vi "SendData_Pub.vi"(8 "error in (no error)":errorcluster, 9 "argument list in":T1[](array[typedef]), 11 "LabVIEW-Python-Interface in":refnum<class "PyLVi.lvclass">) -> (0 "error out":errorcluster, 3 "LabVIEW-Python-Interface out":refnum<class "PyLVi.lvclass">)   [LabVIEW 2016, in "PyLVi.lvlib" / "PyLVi.lvclass"]
uses:
  PyLVi.lvclass
  Controls/ArgumentStructure.ctl
  Controls/DescriptorStructure.ctl
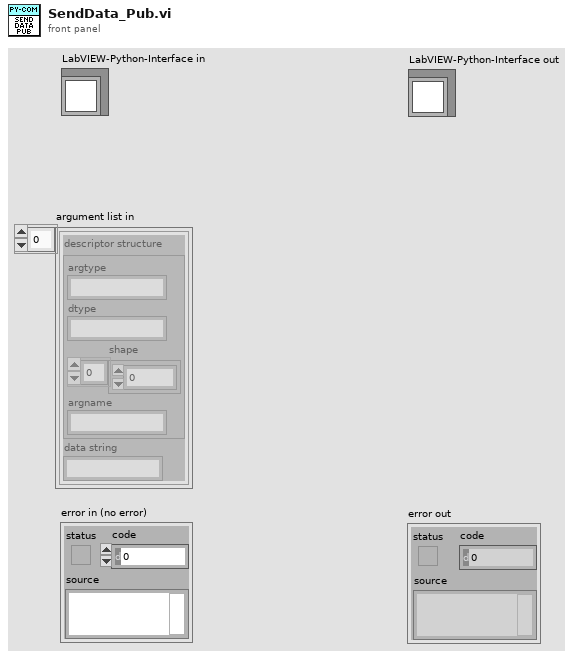
[diagram p1: front panel]
types:
  T1 = typedef "PyLVi.lvlib/PyLVi.lvclass/ArgumentStructure.ctl" = cluster{"descriptor structure":T2, "data string":string}
  T2 = typedef "PyLVi.lvlib/PyLVi.lvclass/DescriptorStructure.ctl" = cluster{"argtype":string, "dtype":string, "shape":u32[], "argname":string}
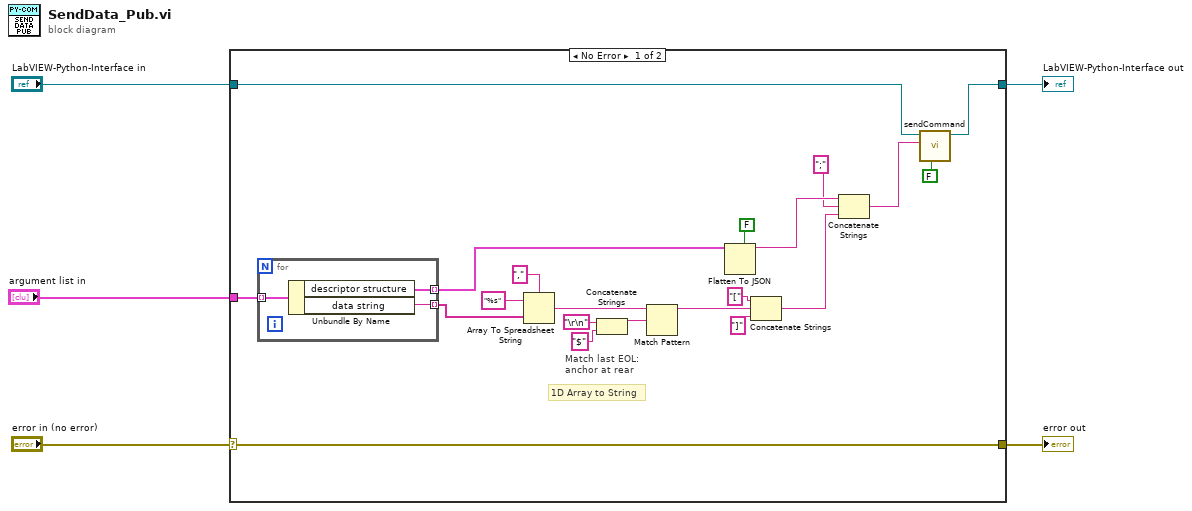
[diagram p0: block diagram]
diagram:
  n1 = case shown="No Error" "error in (no error)" {
    selector: "error in (no error)" -> [w26 w30]
    tunnel: [w26 w30] -> w4
    tunnel: [w24 w31] -> w2
    tunnel: "LabVIEW-Python-Interface in" -> [w25 w31]
    tunnel: "argument list in" -> [w19 _]
    frame No Error {
      # "1D Array to String"
      # "Match last EOL:\nanchor at rear"
      n2 = for {
        tunnel: w19 -> [w29] mode=indexing
        tunnel: [w28] -> w18 mode=indexing
        tunnel: [w27] -> w7 mode=indexing
        n3 = Unbundle By Name(w29) -> ("descriptor structure"=w28:T2, "data string"=w27:string)
      }
      n4 = Array To Spreadsheet String(delimiter (Tab)=",", array=w7, 3:"%s" ("format string")) -> (spreadsheet string=w12:string)
      n5 = Concatenate Strings("\r\n", "$" ("Substring")) -> (w11:string)
      n6 = Match Pattern(string=w12, regular expression=w11) -> (before substring=w6:string)  [unwired: 1 in, 3 out]
      n7 = Flatten To JSON(enable LabVIEW extensions? (T)=FALSE, anything=w18) -> (JSON string=w22:string)  [unwired: 1 in, 1 out]
      n8 = Concatenate Strings("[" ("string"), w6, "]" ("string")) -> (w15:string)
      n9 = Concatenate Strings(w22, ";" ("string"), w15) -> (w20:string)
      n10 = call "sendCommand.vi"("Wait for response (T)"=FALSE, "command"=w20, "LabVIEW-Python-Interface in"=w25) -> ("LabVIEW-Python-Interface out"=w24:refnum<class "PyLVi.lvclass">)  [unwired: 5 in, 3 out]
    }
    frame Error {
    }
  }
  "error out" <- w4
  "LabVIEW-Python-Interface out" <- w2
